vi "EnableRaisingEvent.vi"(8 "错误输入（无错误）":errorcluster, 10 "EnableRaisingEvents":bool, 11 "FilesytemWatcher Ref In":refnum<k24>) -> (0 "错误输出":errorcluster, 3 "FilesytemWatcher Ref Out":refnum<k24>)   [LabVIEW 2012, in "FileSystem Watcher.lvlib"]
uses:
  FileSystem Watcher.lvlib
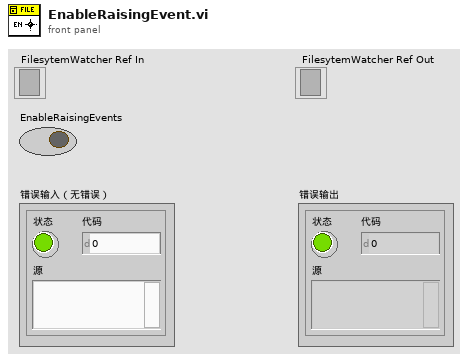
[diagram p1: front panel]
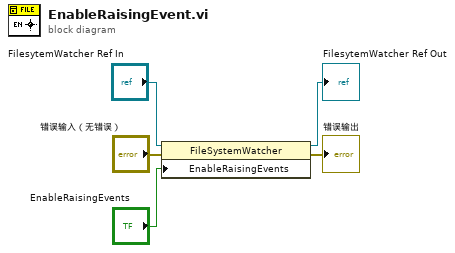
[diagram p0: block diagram]
diagram:
  n1 = property class="FileSystemWatcher"(reference="FilesytemWatcher Ref In", error in="错误输入（无错误）", "EnableRaisingEvents"="EnableRaisingEvents") -> (reference out=→"FilesytemWatcher Ref Out":refnum<k24>, error out=→"错误输出":errorcluster)
